vi "average sensor data.vi"(8 "Numeric":i32, 9 "PixelSize":u16, 10 "Pipe handle":i32, 11 "Device Handle 2":i32) -> (1 "output cluster":cluster{dbl[]}, 2 "XY Graph":cluster{dbl[], dbl[]}(graph) caption="pixel vs A/D Counts", 3 "return type":u16)   [LabVIEW 2013]
uses:
  Users/Ellen/Dropbox/minispec/HamamatsuMinispectrometer/DeveloperTools/ForVisualC++/SampleApl/specu1a.dll
panel:
  in  "default value":u16[](array[numeric])
  in  "default value 2":u16[](array[numeric])
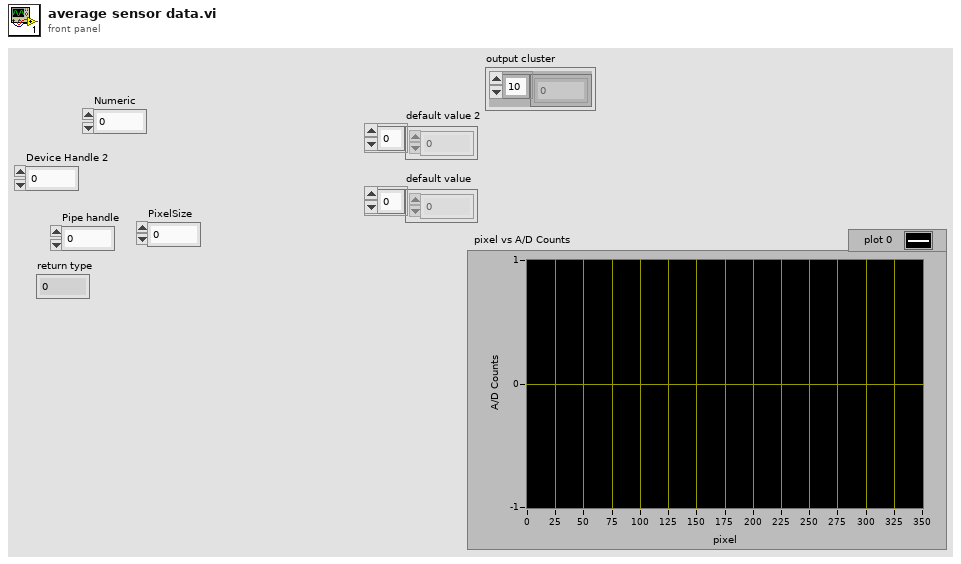
[diagram p1: front panel]
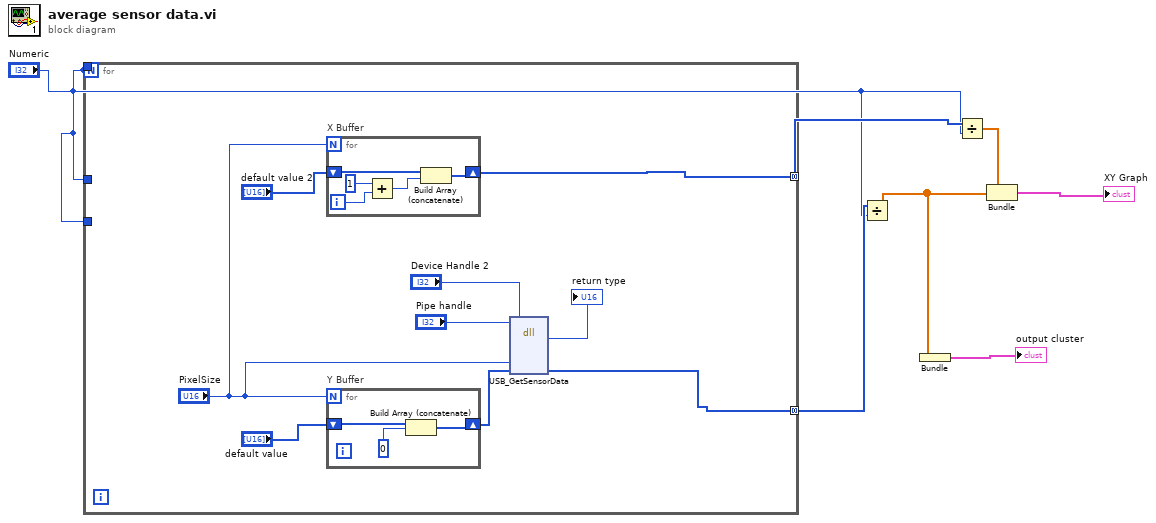
[diagram p0: block diagram]
diagram:
  n1 = for {
    N: "Numeric" -> [_]
    tunnel: "Numeric" -> [_]
    tunnel: "Numeric" -> [_]
    tunnel: "Numeric" -> [_]
    tunnel: [w9] -> w4 mode=concatenating
    tunnel: [w8] -> w6 mode=concatenating
    n2 = for "X Buffer" {
      N: "PixelSize" -> [_]
      shift-right: [w21] -> w9
      shift-left: "default value 2" -> [w20]
      i -> [w19]
      n3 = Add(x=1, y=w19) -> (x+y=w17:i32)
      n4 = Build Array (concatenate)(w20, w17) -> (w21:i32[])
    }
    n5 = for "Y Buffer" {
      N: "PixelSize" -> [_]
      shift-right: [w24] -> w10
      shift-left: "default value" -> [w23]
      n6 = Build Array (concatenate)(w23, 0) -> (w24:i32[])
    }
    n7 = dll-call lib="C:/Users/Ellen/Dropbox/minispec/HamamatsuMinispectrometer/DeveloperTools/ForVisualC++/SampleApl/specu1a.dll" fn="USB_GetSensorData" label="1.0.0 Get sensor data"("Device Handle"="Device Handle 2", "Pipe handle"="Pipe handle", "Pixel size"="PixelSize", "Data buffer"=w10) -> ("return type"=→"return type":u16, "Data buffer"=w8:u16[])  [unwired: 6 in, 2 out]
  }
  n8 = Divide(x=w6, y="Numeric") -> (x/y=w5:dbl[])
  n9 = Bundle(w5) -> (→"output cluster":cluster{dbl[]})  [unwired: 1 in]
  n10 = Divide(x=w4, y="Numeric") -> (x/y=w7:dbl[])
  n11 = Bundle(w7, w5) -> (→"XY Graph":cluster{dbl[], dbl[]})  [unwired: 1 in]
